vi "Validate RaF Custom Device Configuration.vi"(8 "error in (no error)":errorcluster, 11 "Routing and Faulting Custom Device Ref in":T1 format="%.0x") -> (0 "error out":errorcluster, 3 "Routing and Faulting Custom Device Ref out":T1 format="%.0x")   [LabVIEW 2017, in "Routing and Faulting Scripting.lvlib"]
uses:
  Routing and Faulting Scripting.lvlib
  <vilib>/NI Veristand/Custom Device API/Custom Device Item Ref.ctl
  System Explorer/Routing and Faulting System Explorer.lvlib
  NationalInstruments.VeriStand
  <vilib>/NI Veristand/Custom Device API/Custom Device API.lvlib
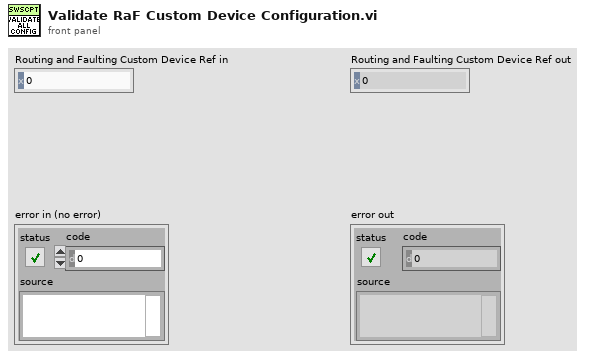
[diagram p1: front panel]
types:
  T1 = typedef "Custom Device API.lvlib/Custom Device Item Ref.ctl" = u64
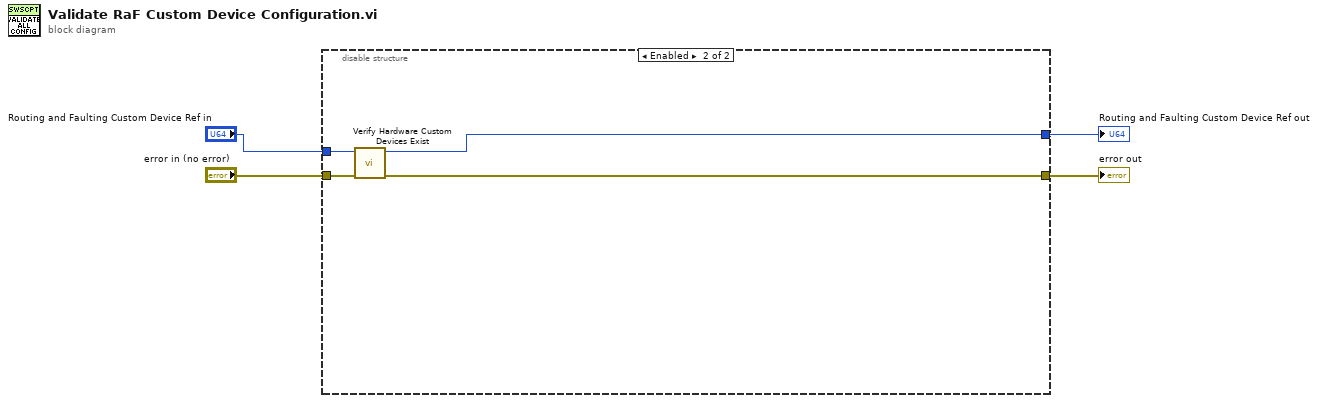
[diagram p0: block diagram]
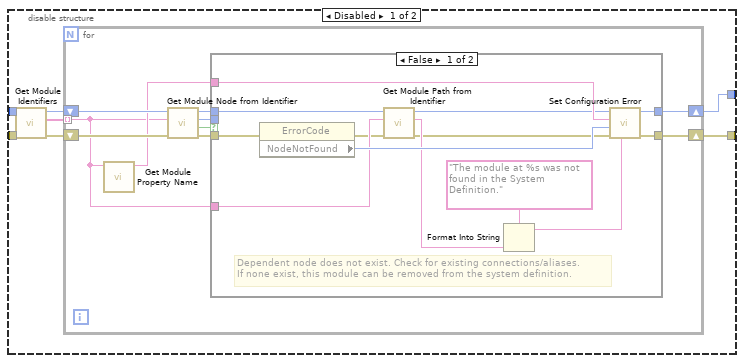
[diagram p2: hidden frame]
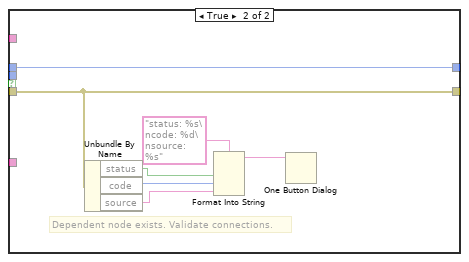
[diagram p3: hidden frame]
diagram:
  n1 = disable-structure shown="Enabled" {
    disable-tunnel: "error in (no error)" -> [w11 w45]
    disable-tunnel: "Routing and Faulting Custom Device Ref in" -> [w10 w44]
    disable-tunnel: [w7 w42] -> w2
    disable-tunnel: [w5 w43] -> w1
    frame Disabled {
      n2 = call "Get Module Identifiers.vi"("error in (no error)"=w11, "Routing and Faulting Ref in"=w10) -> ("error out"=w9:errorcluster, "Module Identifier"=w8:string[], "Routing and Faulting Ref out"=w6:T1)  [unwired: 7 in]
      n3 = for {
        tunnel: w8 -> [w16] mode=indexing
        shift-right: [w20] -> w7
        shift-left: w9 -> [w18]
        shift-right: [w21] -> w5
        shift-left: w6 -> [w19]
        n4 = call "Get Module Property Name.vi"("Module ID"=w16) -> ("Module Property Name"=w17:string)  [unwired: 10 in]
        n5 = call "Get Module Node from Identifier.vi"("error in (no error)"=w18, "Module identifier"=w16, "Routing and Faulting Ref in"=w19) -> ("error out"=w12:errorcluster, "Found"=w15:bool, "Module Node"=w14:T1, "Routing and Faulting Ref out"=w13:T1)  [unwired: 5 in]
        n6 = case shown="False" w15 {
          tunnel: w12 -> [w34 w39]
          tunnel: [w33 w41] -> w21
          tunnel: [w32 w39] -> w20
          tunnel: w17 -> [w31 _]
          tunnel: w16 -> [w29 _]
          tunnel: w14 -> [_ _]
          tunnel: w13 -> [w24 w41]
          frame False {
            # "Dependent node does not exist. Check for existing connections/aliases.\nIf none exist, this module can be removed from the system definition."
            n7 = property class="ErrorCode"(error in=w34) -> (error out=w23:errorcluster, "NodeNotFound"=w30:i32)  [unwired: 1 in, 1 out]
            n8 = call "Get Module Path from Identifier.vi"("error in (no error)"=w23, "Module identifier"=w29, "Routing and Faulting Ref in"=w24) -> ("error out"=w22:errorcluster, "Module path"=w27:string, "Routing and Faulting Ref out"=w26:T1)  [unwired: 6 in]
            n9 = Format Into String(format string="The module at %s was not found in the System Definition." ("Message"), w27) -> (resulting string=w25:string)  [unwired: 2 in, 1 out]
            n10 = call "Set Configuration Error.vi"("Message"=w25, "error in (no error)"=w22, "NationalInstruments.VeriStand.ErrorCode"=w30, "Key"=w31, "Item Ref in"=w26) -> ("error out"=w32:errorcluster, "Item Ref out"=w33:T1)  [unwired: 5 in]
          }
          frame True {
            # "Dependent node exists. Validate connections."
            n11 = Unbundle By Name(w39) -> ("status"=w38:bool, "code"=w36:i32, "source"=w35:string)
            n12 = Format Into String(format string="status: %s\ncode: %d\nsource: %s", w38, w36, w35) -> (resulting string=w37:string)  [unwired: 2 in, 1 out]
            n13 = One Button Dialog(message=w37) -> ()  [unwired: 1 in, 1 out]
          }
        }
      }
    }
    frame Enabled {
      n14 = call "Verify Hardware Custom Devices Exist.vi"("error in (no error)"=w45, "Routing and Faulting Custom Device Ref in"=w44) -> ("error out"=w42:errorcluster, "Routing and Faulting Custom Device Ref out"=w43:T1)  [unwired: 8 in]
    }
  }
  "Routing and Faulting Custom Device Ref out" <- w1
  "error out" <- w2
